vi "MeasAction.vi"(8 "error in (no error)":errorcluster caption="entrée d'erreur (pas d'erreur)", 9 "CurvePointIndex":i32, 10 "AllPointIndex":i32, 11 "GenData In":refnum<class "EG_G5210.lvclass"> caption="DNL_LabVIEW Object in") -> (0 "error out":errorcluster caption="sortie d'erreur", 2 "MeasDatOut":dbl[](array[numeric]), 3 "GenData Out":refnum<class "EG_G5210.lvclass"> caption="DNL_LabVIEW Object out")   [LabVIEW 2010, in "EG_G5210.lvclass"]
uses:
  EG_G5210.lvclass
  EG_G5210.lvclass/EG_G5210.ctl
  BaseDevice/BaseDevice.lvclass
  <userlib>/GenProg/WritebyWeakRefBool.vi
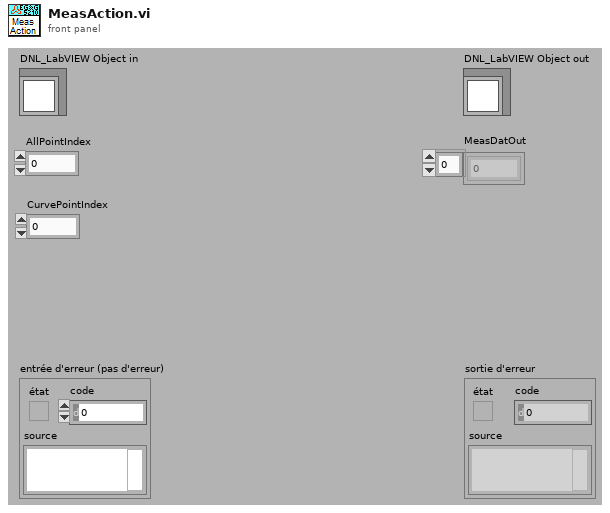
[diagram p1: front panel]
types:
  T1 = enum16{"X Output", "Y Output", "X and Y Output", "Mag", "Phase", "Mag & Phase", "X,Y,Mag & Phase", "Noise", "Aux In 1", "Aux In 2", "Aux In 3", "Aux In 4"}
  T2 = typedef "EG_G5210.lvclass/EG_G5210_Func.ctl" = enum16{"Read X & Y (V)", "Read Mag & Phase (V,°)", "Read X, Y, Mag & Phase (V,V,V,°)", "Read ADC Ch1 (V)", "Read ADC Ch2 (V)"}
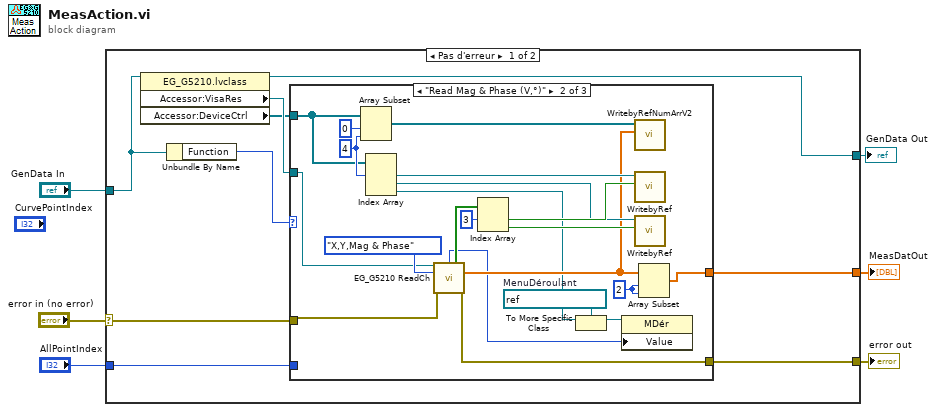
[diagram p0: block diagram]
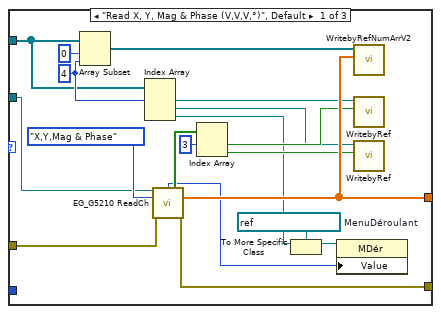
[diagram p2: hidden frame]
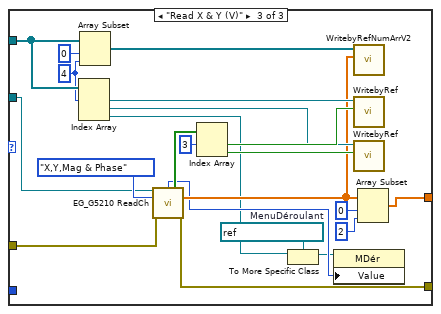
[diagram p3: hidden frame]
diagram:
  n1 = case shown="Pas d'erreur" "error in (no error)" {
    selector: "error in (no error)" -> [w12 w78]
    tunnel: "GenData In" -> [w10 w79]
    tunnel: [w9 w79] -> w4
    tunnel: "AllPointIndex" -> [w15 _]
    tunnel: [w14 w78] -> w2
    tunnel: [w13 _] -> w1
    frame No Error {
      n2 = property class="EG_G5210.lvclass"(reference=w10) -> (reference out=w9:refnum<class "EG_G5210.lvclass">, "Accessor:VisaRes"=w8:refnum<visa-resource-name>, "Accessor:DeviceCtrl"=w7:refnum<vi>[])  [unwired: 1 in, 1 out]
      n3 = Unbundle By Name(w10) -> ("Function"=w11:T2)
      n4 = case shown="\"Read Mag & Phase (V,°)\"" w11 {
        tunnel: w15 -> [_ _ _]
        tunnel: [w28 w50 w72] -> w14
        tunnel: [w30 w41 w64] -> w13
        tunnel: w12 -> [w34 w55 w77]
        tunnel: w8 -> [w32 w53 w75]
        tunnel: w7 -> [w20 w42 w65]
        frame "Read X, Y, Mag & Phase (V,V,V,°)", Default {
          w17 = refnum<vi> refnum  # MenuDéroulant
          w27 = 4 ("longueur")
          n5 = Array Subset(array=w20, index=0 ("indice"), length=w27) -> (w29:refnum<vi>[])
          n6 = Index Array(array=w20, index #1=w27) -> (element #1=w24:refnum<vi>, element #2=w22:refnum<vi>, element #3=w19:refnum<vi>)  [unwired: 2 in]
          n7 = call <userlib>:"EG_G5210 ReadCh.vi"("VISA Rsrc"=w32, "Channel"=T1."X,Y,Mag & Phase", "error in (no error)"=w34) -> ("Sensitivity"=w16:u16, "Status Byte"=w26:bool[], "Outputs"=w30:dbl[], "error out"=w28:errorcluster)  [unwired: 5 in, 4 out]
          n8 = Index Array(array=w26, index #1=3 ("indice")) -> (element #1=w23:bool, element #2=w21:bool)  [unwired: 1 in]
          n9 = To More Specific Class(target class=w17, reference=w19) -> (specific class reference=w18:refnum<vi>)  [unwired: 1 in, 1 out]
          n10 = property class="MDér"(reference=w18, "Value"=w16) -> ()  [unwired: 1 in, 2 out]
          n11 = call <userlib>:"WritebyRefNumArrV2.vi"("Tableau"=w30, "Ctrl Ref"=w29) -> ()  [unwired: 9 in, 1 out]
          n12 = call-poly <userlib>:"WritebyRef.vi"("Valeur"=w23, "Control Ref"=w24) -> ()  [unwired: 9 in, 1 out]
          n13 = call-poly <userlib>:"WritebyRef.vi"("Valeur"=w21, "Control Ref"=w22) -> ()  [unwired: 9 in, 1 out]
        }
        frame "Read Mag & Phase (V,°)" {
          w36 = refnum<vi> refnum  # MenuDéroulant
          w39 = 2 ("indice")
          w49 = 4 ("longueur")
          n14 = Array Subset(array=w42, index=0 ("indice"), length=w49) -> (w51:refnum<vi>[])
          n15 = Index Array(array=w42, index #1=w49) -> (element #1=w46:refnum<vi>, element #2=w44:refnum<vi>, element #3=w37:refnum<vi>)  [unwired: 2 in]
          n16 = call <userlib>:"EG_G5210 ReadCh.vi"("VISA Rsrc"=w53, "Channel"=T1."X,Y,Mag & Phase", "error in (no error)"=w55) -> ("Sensitivity"=w35:u16, "Status Byte"=w48:bool[], "Outputs"=w40:dbl[], "error out"=w50:errorcluster)  [unwired: 5 in, 4 out]
          n17 = Index Array(array=w48, index #1=3 ("indice")) -> (element #1=w45:bool, element #2=w43:bool)  [unwired: 1 in]
          n18 = To More Specific Class(target class=w36, reference=w37) -> (specific class reference=w38:refnum<vi>)  [unwired: 1 in, 1 out]
          n19 = property class="MDér"(reference=w38, "Value"=w35) -> ()  [unwired: 1 in, 2 out]
          n20 = call <userlib>:"WritebyRefNumArrV2.vi"("Tableau"=w40, "Ctrl Ref"=w51) -> ()  [unwired: 9 in, 1 out]
          n21 = call-poly <userlib>:"WritebyRef.vi"("Valeur"=w45, "Control Ref"=w46) -> ()  [unwired: 9 in, 1 out]
          n22 = call-poly <userlib>:"WritebyRef.vi"("Valeur"=w43, "Control Ref"=w44) -> ()  [unwired: 9 in, 1 out]
          n23 = Array Subset(array=w40, index=w39, length=w39) -> (w41:dbl[])
        }
        frame "Read X & Y (V)" {
          w57 = refnum<vi> refnum  # MenuDéroulant
          w60 = 4 ("longueur")
          n24 = Index Array(array=w65, index #1=w60) -> (element #1=w69:refnum<vi>, element #2=w67:refnum<vi>, element #3=w56:refnum<vi>)  [unwired: 2 in]
          n25 = Array Subset(array=w65, index=0 ("indice"), length=w60) -> (w73:refnum<vi>[])
          n26 = call <userlib>:"EG_G5210 ReadCh.vi"("VISA Rsrc"=w75, "Channel"=T1."X,Y,Mag & Phase", "error in (no error)"=w77) -> ("Sensitivity"=w59:u16, "Status Byte"=w71:bool[], "Outputs"=w63:dbl[], "error out"=w72:errorcluster)  [unwired: 5 in, 4 out]
          n27 = Index Array(array=w71, index #1=3 ("indice")) -> (element #1=w68:bool, element #2=w66:bool)  [unwired: 1 in]
          n28 = To More Specific Class(target class=w57, reference=w56) -> (specific class reference=w58:refnum<vi>)  [unwired: 1 in, 1 out]
          n29 = property class="MDér"(reference=w58, "Value"=w59) -> ()  [unwired: 1 in, 2 out]
          n30 = call <userlib>:"WritebyRefNumArrV2.vi"("Tableau"=w63, "Ctrl Ref"=w73) -> ()  [unwired: 9 in, 1 out]
          n31 = call-poly <userlib>:"WritebyRef.vi"("Valeur"=w68, "Control Ref"=w69) -> ()  [unwired: 9 in, 1 out]
          n32 = call-poly <userlib>:"WritebyRef.vi"("Valeur"=w66, "Control Ref"=w67) -> ()  [unwired: 9 in, 1 out]
          n33 = Array Subset(array=w63, index=0 ("indice"), length=2 ("indice")) -> (w64:dbl[])
        }
      }
    }
    frame Error {
    }
  }
  "error out" <- w2
  "GenData Out" <- w4
  "MeasDatOut" <- w1
